vi "initialize assembly lists.vi"(4 "output dictionary":refnum<class "data dictionary.lvclass">, 6 "input dictionary":refnum<class "data dictionary.lvclass">, 8 "error in":errorcluster, 10 "EthernetIP configuration in":refnum<class "EIP Tags Configuration.lvclass">, 11 "EthernetIP runtime in":refnum<class "EIP Tags Runtime.lvclass">) -> (0 "error out":errorcluster, 3 "EthernetIP runtime out":refnum<class "EIP Tags Runtime.lvclass">)   [LabVIEW 2013, in "EIP Tags Runtime.lvclass"]
uses:
  EIP Tags Runtime.lvclass
  configuration/EIP Tags Configuration.lvclass
  <vilib>/NI/Tag Bus/dictionary/data dictionary.lvclass
  <vilib>/ethernetip/ethernetip.llb/ethernetip.ctl
  assembly data spec.ctl
  conversion specification.ctl
  <vilib>/NI/Tag Bus/tag/Data Type.ctl
  configuration/EIP Tags Configuration.lvclass/EIP Tags Configuration.ctl
  <vilib>/ethernetip/ethernetip.llb/EthernetIPAssemblyType.ctl
  channel/EIP Tags Channel.lvclass/EIP Tags Channel.ctl
  <vilib>/NI/Tag Bus/tag/tag descriptor.lvclass/tag descriptor.ctl
  <vilib>/NI/Tag Bus Module Framework/channel/TBM channel.lvclass/TBM channel.ctl
  EIP Tags Runtime.lvclass/EIP Tags Runtime.ctl
  channel/Read Instance ID.vi
  <vilib>/NI/Tag Bus/tag/read tag name.vi
  <vilib>/NI/Tag Bus Module Framework/channel/Read channel classification.vi
  <vilib>/NI/Tag Bus/tag/read data type.vi
  channel/Read byte index.vi
  channel/Read subindex.vi
  configuration/Read assemblies.vi
  configuration/read eip channels.vi
  channel/EIP Tags Channel.lvclass
  <vilib>/NI/Tag Bus/tag/tag descriptor.lvclass
  <vilib>/ethernetip/ethernetip.lvlib
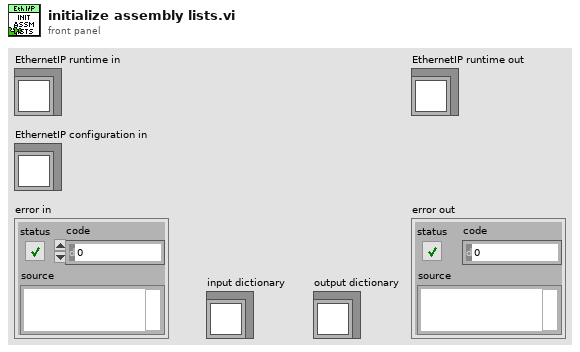
[diagram p1: front panel]
types:
  T1 = typedef "EIP Tags Runtime.lvclass/assembly data spec.ctl" = cluster{"Instance ID":u32, "specification":T2[], "big endian?":bool}
  T2 = typedef "EIP Tags Runtime.lvclass/conversion specification.ctl" = cluster{"data type":T3, "data index":i32, "byte index":i32, "subindex":i32}
  T3 = typedef "tag bus.lvlib/tag descriptor.lvclass/Data Type.ctl" = enum16{"Double", "Single", "I64", "I32", "I16", "I8", "U64", "U32", "U16", "U8", "Boolean", "String", "Array of Double", "Array of Single", "Array of I64", "Array of I32", "Array of I16", "Array of I8", "Array of U64", "Array of U32", "Array of U16", "Array of U8", "Array of Boolean", "Array of String"}
  T4 = typedef "ethernetip.lvlib/ethernetip.ctl" = refnum<k21>
  T5 = typedef "EthernetIP configuration.lvclass/assembly definition.ctl" = cluster{"name":string, "Instance ID":u32, "Type":T6, "Size (bytes)":u32, "big endian?":bool}
  T6 = typedef "EthernetIP configuration.lvclass/assembly type.ctl" = enum32{"Producing", "Consuming"}
  T7 = typedef "ethernetip.lvlib/EthernetIPAssemblyType.ctl" = enum16{"Producing", "Consuming", "Configuration"}
  T8 = typedef "TBM channel.lvclass/channel classification.ctl" = enum16{"input data", "output data", "processing parameter", "processing result"}
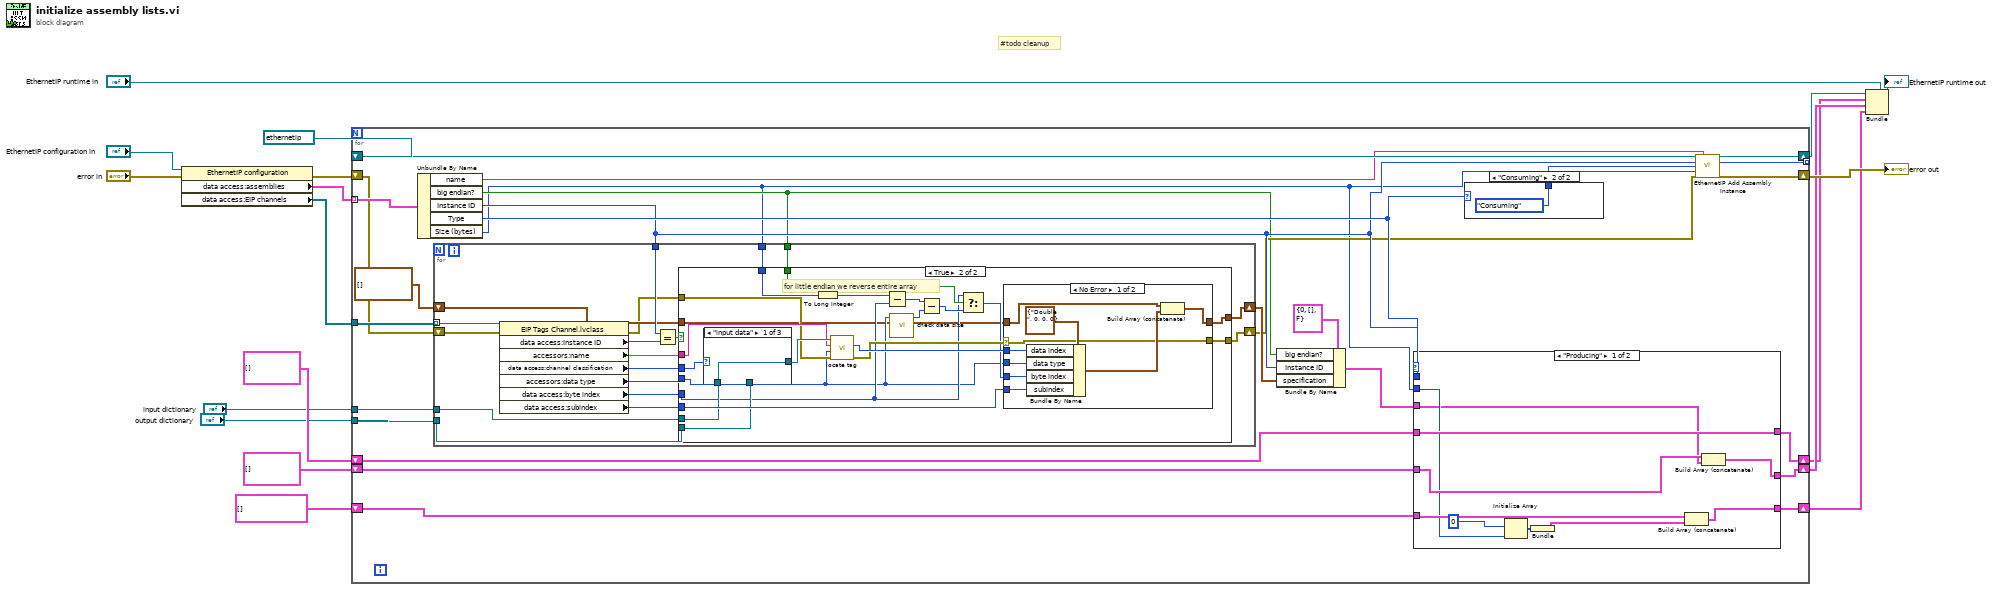
[diagram p0: block diagram]
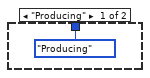
[diagram p6: hidden frame]
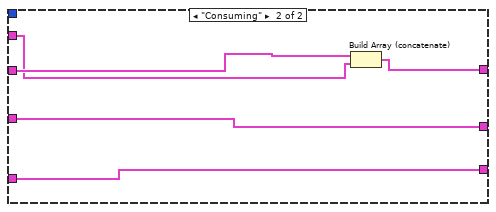
[diagram p7: hidden frame]
diagram:
  # "#todo cleanup"
  n1 = property class="EthernetIP configuration"(reference="EthernetIP configuration in", error in="error in") -> (error out=w14:errorcluster, "data access:assemblies"=w17:T5[], "data access:EIP channels"=w18:refnum<class "EIP Tags Channel.lvclass">[])  [unwired: 1 out]
  n2 = for {
    shift-right: [w44] -> w11
    shift-left: w14 -> [w24]
    shift-right: [w43] -> w13
    shift-left: T4 "Default" ("Session in") -> [w42]
    tunnel: w17 -> [w41] mode=indexing
    tunnel: [w39] -> _ mode=indexing
    tunnel: w18 -> [w30]
    shift-right: [w31] -> w3
    shift-left: T1[] [] ("output assemblies") -> [w32]
    shift-right: [w36] -> w4
    shift-left: T1[] [] ("output assemblies") -> [w35]
    shift-right: [w33] -> w5
    shift-left: cluster{"output allocation":u8[]}[] [] ("output allocations") -> [w34]
    tunnel: "input dictionary" -> [w22]
    tunnel: "output dictionary" -> [w21]
    n3 = Unbundle By Name(w41) -> ("name"=w40:string, "big endian?"=w20:bool, "Instance ID"=w27:u32, "Type"=w38:T6, "Size (bytes)"=w19:u32)
    n4 = for {
      tunnel: w30 -> [w62] mode=indexing
      tunnel: w27 -> [w61]
      shift-right: [w60] -> w26
      shift-left: T2[] [] ("specification") -> [w59]
      shift-right: [w47] -> w23
      shift-left: w24 -> [w53]
      tunnel: w22 -> [w51]
      tunnel: w21 -> [w50]
      tunnel: w20 -> [w46]
      tunnel: w19 -> [w45]
      n5 = property class="EIP Tags Channel.lvclass"(reference=w62, error in=w53) -> (error out=w48:errorcluster, "data access:Instance ID"=w54:u32, "accessors:name"=w49:string, "data access:channel classification"=w52:T8, "accessors:data type"=w55:T3, "data access:byte index"=w56:i32, "data access:subindex"=w57:i32)  [unwired: 1 out]
      n6 = Equal?(x=w61, y=w54) -> (x = y?=w58:bool)
      n7 = case shown="True" w58 {
        tunnel: [w64 w85] -> w60
        tunnel: w59 -> [w64 w65]
        tunnel: w57 -> [_ w84]
        tunnel: w56 -> [_ w68]
        tunnel: w55 -> [_ w67]
        tunnel: w52 -> [_ w83]
        tunnel: w51 -> [_ w82]
        tunnel: w50 -> [_ w81]
        tunnel: w49 -> [_ w79]
        tunnel: w48 -> [w63 w78]
        tunnel: [w63 w75] -> w47
        tunnel: w46 -> [_ w72]
        tunnel: w45 -> [_ w74]
        frame False {
        }
        frame True {
          # "for little endian we reverse entire array"
          n8 = case shown="\"input data\"" w83 {
            tunnel: w82 -> [w86 _ _]
            tunnel: w81 -> [_ _ w87]
            tunnel: [w86 _ w87] -> w80
            frame "input data" {
            }
            frame Default {
            }
            frame "output data" {
            }
          }
          n9 = To Long Integer(number=w74) -> (32bit integer=w69:i32)
          n10 = call <vilib>:"locate tag.vi"("error in"=w78, "data type"=w67, "name"=w79, "data dictionary in"=w80) -> ("error out"=w76:errorcluster, "index"=w77:i32)  [unwired: 5 in, 1 out]
          n11 = Subtract(x=w69, y=w68) -> (x-y=w73:i32)
          n12 = call "check data size.vi"("data type"=w67) -> ("bytes"=w66:i32)  [unwired: 10 in]
          n13 = Subtract(x=w73, y=w66) -> (x-y=w71:i32)
          n14 = Select(t=w68, s=w72, f=w71) -> (s? t:f=w70:i32)
          n15 = case shown="No Error" w76 {
            selector: w76 -> [w88 w97]
            tunnel: [w90 w98] -> w85
            tunnel: w65 -> [w91 w98]
            tunnel: w84 -> [w95 _]
            tunnel: w70 -> [w94 _]
            tunnel: w67 -> [w93 _]
            tunnel: w77 -> [w89 _]
            tunnel: [w88 w97] -> w75
            frame No Error {
              n16 = Bundle By Name(cluster=T2 {"data type"=enum."Double", "data index"=0, "byte index"=0, "subindex"=0} ("specification"), "data index"=w89, "data type"=w93, "byte index"=w94, "subindex"=w95) -> (w92:T2)
              n17 = Build Array (concatenate)(w91, w92) -> (w90:T2[])
            }
            frame Error {
            }
          }
        }
      }
    }
    n18 = Bundle By Name(cluster=T1 {"Instance ID"=0, "specification"=[], "big endian?"=FALSE} ("assembly data spec"), "big endian?"=w20, "Instance ID"=w27, "specification"=w26) -> (w25:T1)
    n19 = case shown="\"Producing\"" w38 {
      tunnel: w27 -> [_ _]
      tunnel: w19 -> [w105 _]
      tunnel: [w110 w115] -> w36
      tunnel: w35 -> [w109 w115]
      tunnel: w34 -> [w107 w114]
      tunnel: [w108 w114] -> w33
      tunnel: w32 -> [w106 w113]
      tunnel: [w106 w112] -> w31
      tunnel: w25 -> [w101 w111]
      frame "Producing" {
        n20 = Initialize Array(u8 0, w105) -> (w103:u8[])
        n21 = Bundle(w103) -> (w102:cluster{u8[]})  [unwired: 1 in]
        n22 = Build Array (concatenate)(w107, w102) -> (w108:cluster{"output allocation":u8[]}[])
        n23 = Build Array (concatenate)(w109, w101) -> (w110:T1[])
      }
      frame "Consuming" {
        n24 = Build Array (concatenate)(w113, w111) -> (w112:T1[])
      }
    }
    n25 = case shown="\"Consuming\"" w38 {
      tunnel: [EthernetIPAssemblyType."Producing" ("Type") EthernetIPAssemblyType."Consuming" ("Type")] -> w37
      frame "Producing" {
      }
      frame "Consuming" {
      }
    }
    n26 = call <vilib>:"EthernetIP Add Assembly Instance.vi"("Session in"=w42, "Name (optional)"=w40, "Instance ID in"=w27, "Type"=w37, "Size (bytes)"=w19, "error in"=w23) -> ("Session out"=w43:T4, "Instance ID out"=w39:u32, "error out"=w44:errorcluster)  [unwired: 7 in]
  }
  "error out" <- w11
  n27 = Bundle(cluster="EthernetIP runtime in", w13, w3, w4, w5) -> (→"EthernetIP runtime out":refnum<class "EIP Tags Runtime.lvclass">)
